vi "Write CAN Data in tdms.vi"(7 "Commnad":T1, 8 "error in (no error)":errorcluster, 11 "CAN Frame":string[][](array[string])) -> (0 "error out":errorcluster)   [LabVIEW 2016, in "CAN.lvlib"]
uses:
  CAN.lvlib
  User Interface/Log Data Command.ctl
  User Interface/Create Path Command.ctl
  User Interface/User Interface.lvlib
panel:
  in  "Channel name":string[](array[string])
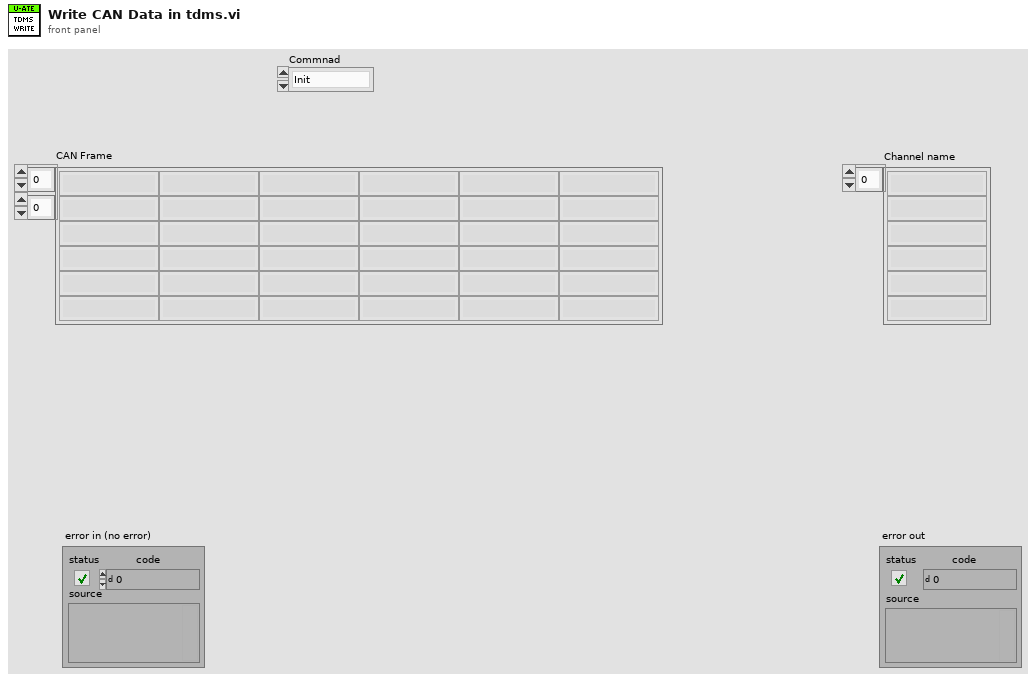
[diagram p1: front panel]
types:
  T1 = typedef "User Interface.lvlib/Log Data Command.ctl" = enum16{"Init", "Read", "Write", "Close"}
  T2 = typedef "User Interface.lvlib/Create Path Command.ctl" = enum16{"Authentication", "Hardware", "Configuration", "Calibration", "Instrument", "Test Description", "Serial Data", "ARINC Data", "CAN Data", "Data", "Report", "Action log", "Error Log"}
  T3 = enum16{"open", "open or create", "create or replace", "create", "open (read-only)"}
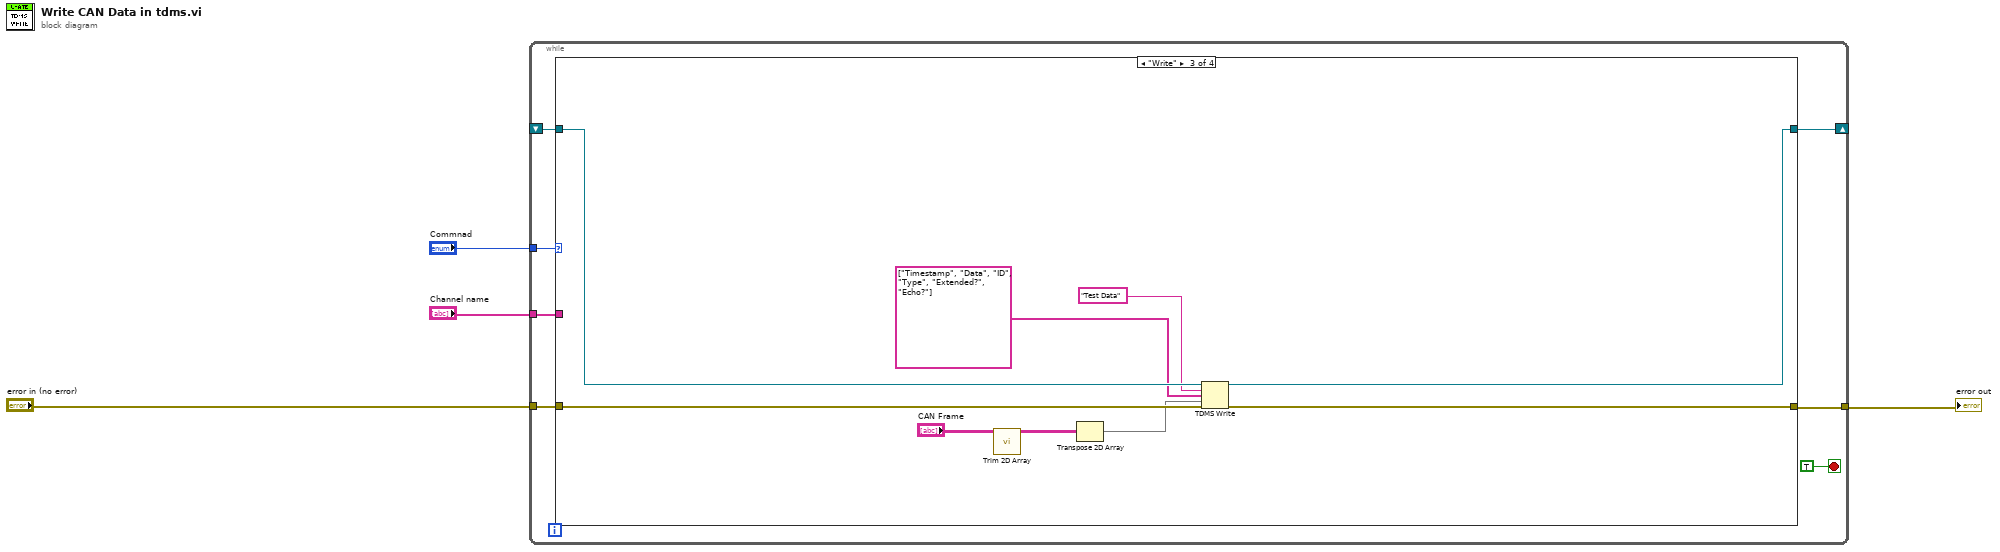
[diagram p0: block diagram]
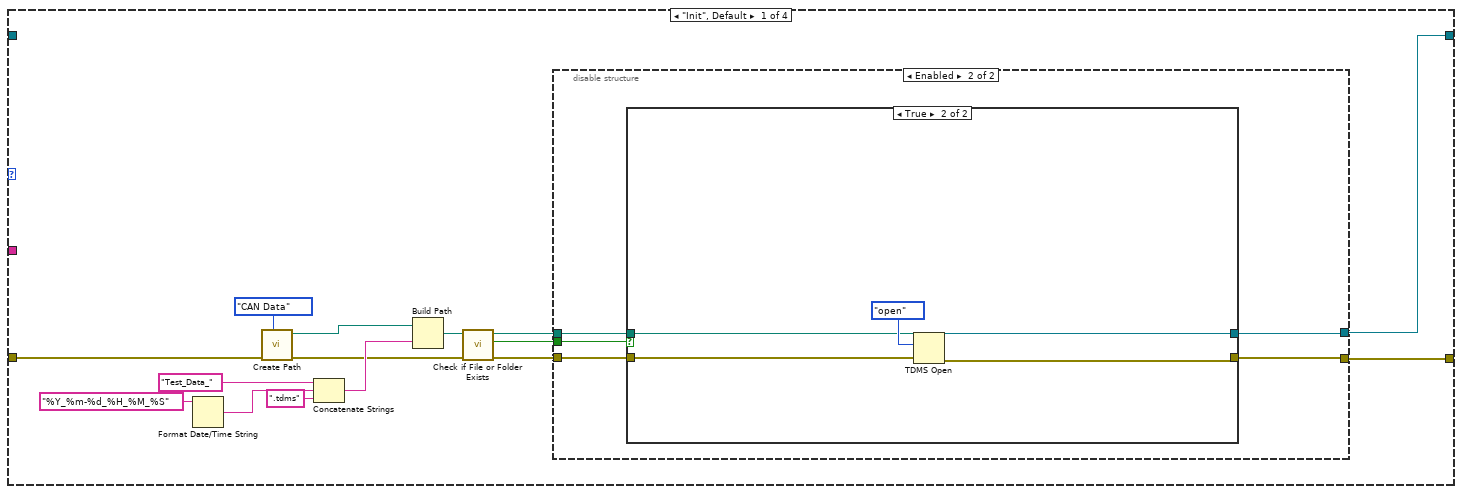
[diagram p2: hidden frame]
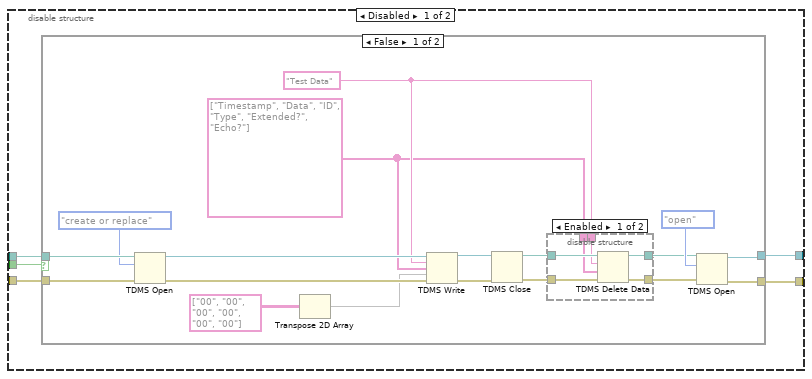
[diagram p3: hidden frame]
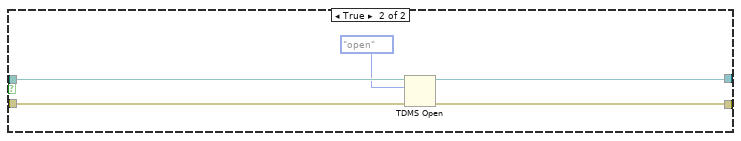
[diagram p5: hidden frame]
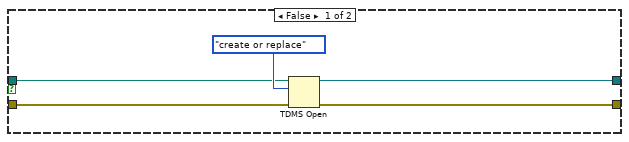
[diagram p6: hidden frame]
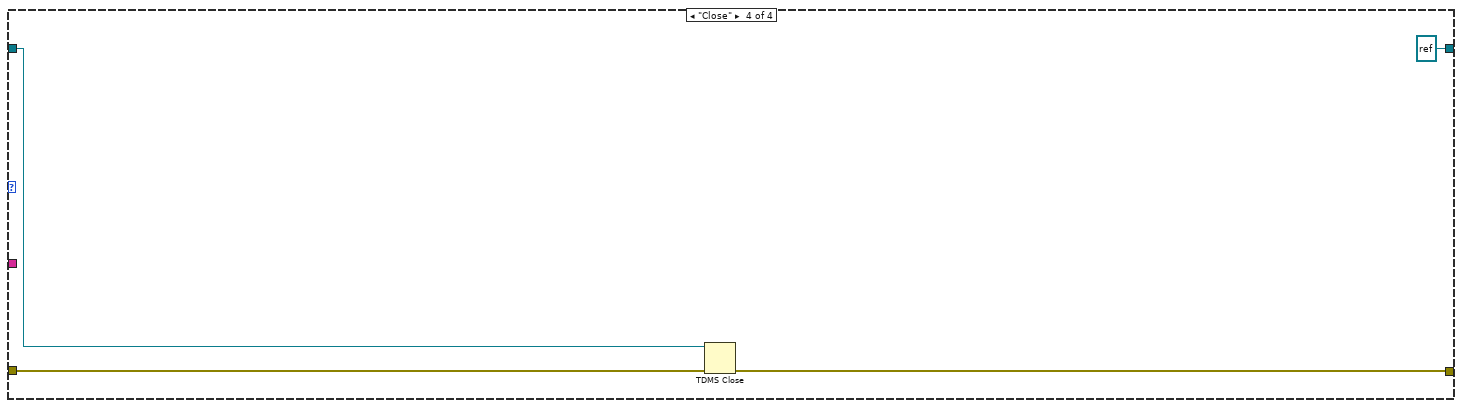
[diagram p8: hidden frame]
diagram:
  n1 = while {
    tunnel: "error in (no error)" -> [w10]
    tunnel: "Commnad" -> [w9]
    tunnel: [w8] -> w2
    shift-right: [w7] -> _
    shift-left: _ -> [w6]
    tunnel: "Channel name" -> [w5]
    stop <- TRUE stop-if-true
    n2 = case shown="\"Write\"" w9 {
      tunnel: w10 -> [w26 w78 w88 w92]
      tunnel: [w13 w78 w85 w91] -> w8
      tunnel: [w12 w79 w86 refnum<k34> refnum ("tdms file out")] -> w7
      tunnel: w6 -> [_ w79 w87 w90]
      tunnel: w5 -> [_ _ _ _]
      frame "Init", Default {
        n3 = Format Date/Time String(time format string (%c)="%Y_%m-%d_%H_%M_%S") -> (date/time string=w18:string)  [unwired: 2 in]
        n4 = call "Create Path.vi"("Path Command"=Create_Path_Command."CAN Data", "error in (no error)"=w26) -> ("error out"=w14:errorcluster, "created path"=w20:path)  [unwired: 8 in]
        n5 = Concatenate Strings("Test_Data_" ("string"), w18, ".tdms" ("string")) -> (w16:string)
        n6 = Build Path(base path=w20, name or relative path=w16) -> (appended path=w15:path)
        n7 = call <vilib>:"Check if File or Folder Exists.vi"("error in (no error)"=w14, "path"=w15) -> ("error out"=w24:errorcluster, "file or folder exists?"=w23:bool, "dup path"=w22:path)  [unwired: 7 in]
        n8 = disable-structure shown="Enabled" {
          disable-tunnel: w24 -> [w31 w66]
          disable-tunnel: w23 -> [w30 w67]
          disable-tunnel: w22 -> [w29 w63]
          disable-tunnel: [w28 w64] -> w13
          disable-tunnel: [w27 w65] -> w12
          frame Disabled {
            n9 = case shown="False" w30 {
              tunnel: w31 -> [w48 w62]
              tunnel: w29 -> [w49 w61]
              tunnel: [w41 w59] -> w28
              tunnel: [w42 w60] -> w27
              frame False {
                w32 = string[] ["Timestamp", "Data", "ID", "Type", "Extended?", "Echo?"]
                w33 = "Test Data"
                n10 = TDMS Open(8:w48, 10:T3."create or replace" ("operation (0:open)"), 11:w49) -> (0:w46:errorcluster, 3:w45:refnum<k34>)  [unwired: 4 in]
                n11 = Transpose 2D Array(2D array=string[][] [["00", "00", "00", "00", "00", "00"]]) -> (transposed array=w38:string[][])
                n12 = TDMS Write(0:w45, 5:w33, 7:w32, 9:w38, 11:w46) -> (4:w44:refnum<k34>, 15:w43:errorcluster)  [unwired: 1 in, 2 out]
                n13 = TDMS Close(8:w43, 11:w44) -> (0:w37:errorcluster, 3:w36:path)
                n14 = disable-structure shown="Enabled" {
                  disable-tunnel: w37 -> [w55 w56]
                  disable-tunnel: w36 -> [w54 w57]
                  disable-tunnel: [w53 w57] -> w35
                  disable-tunnel: [w52 w56] -> w34
                  disable-tunnel: w33 -> [w51 _]
                  disable-tunnel: w32 -> [w50 _]
                  frame Enabled {
                    n15 = TDMS Delete Data(8:w55, 9:w50, 10:w51, 11:w54) -> (0:w52:errorcluster, 3:w53:path)  [unwired: 3 in]
                  }
                  frame Disabled {
                  }
                }
                n16 = TDMS Open(8:w34, 10:T3."open" ("operation (0:open)"), 11:w35) -> (0:w41:errorcluster, 3:w42:refnum<k34>)  [unwired: 4 in]
              }
              frame True {
                n17 = TDMS Open(8:w62, 10:T3."open" ("operation (0:open)"), 11:w61) -> (0:w59:errorcluster, 3:w60:refnum<k34>)  [unwired: 4 in]
              }
            }
          }
          frame Enabled {
            n18 = case shown="True" w67 {
              tunnel: w66 -> [w71 w75]
              tunnel: [w70 w74] -> w65
              tunnel: [w69 w73] -> w64
              tunnel: w63 -> [w68 w76]
              frame False {
                n19 = TDMS Open(8:w71, 10:T3."create or replace" ("operation (0:open)"), 11:w68) -> (0:w69:errorcluster, 3:w70:refnum<k34>)  [unwired: 4 in]
              }
              frame True {
                n20 = TDMS Open(8:w75, 10:T3."open" ("operation (0:open)"), 11:w76) -> (0:w73:errorcluster, 3:w74:refnum<k34>)  [unwired: 4 in]
              }
            }
          }
        }
      }
      frame "Read" {
      }
      frame "Write" {
        n21 = call "Trim 2D Array.vi"("Data in"="CAN Frame") -> ("Data out"=w82:string[][])  [unwired: 10 in]
        n22 = Transpose 2D Array(2D array=w82) -> (transposed array=w80:string[][])
        n23 = TDMS Write(0:w87, 5:"Test Data", 7:string[] ["Timestamp", "Data", "ID", "Type", "Extended?", "Echo?"], 9:w80, 11:w88) -> (4:w86:refnum<k34>, 15:w85:errorcluster)  [unwired: 1 in, 2 out]
      }
      frame "Close" {
        n24 = TDMS Close(8:w92, 11:w90) -> (0:w91:errorcluster)  [unwired: 1 out]
      }
    }
  }
  "error out" <- w2
